vi "Memory Usage.vi"(8 "error in (no error)":errorcluster, 11 "System Status Actor in":refnum<class "System Status Actor.lvclass">) -> (0 "error out":errorcluster, 3 "System Status Actor out":refnum<class "System Status Actor.lvclass">)   [LabVIEW 2020, in "RTAF.lvlib" / "System Status Actor.lvclass"]
uses:
  System Status Actor.lvclass
  System Status Actor.lvclass/System Status Actor.ctl
panel:
  out "Total [MB]":dbl
  out "Used [MB]":dbl
  out "cat /proc/$(pidof lvrt)/status | grep RSS":string
  out "Free [MB]":dbl
  out "/proc/meminfo":string
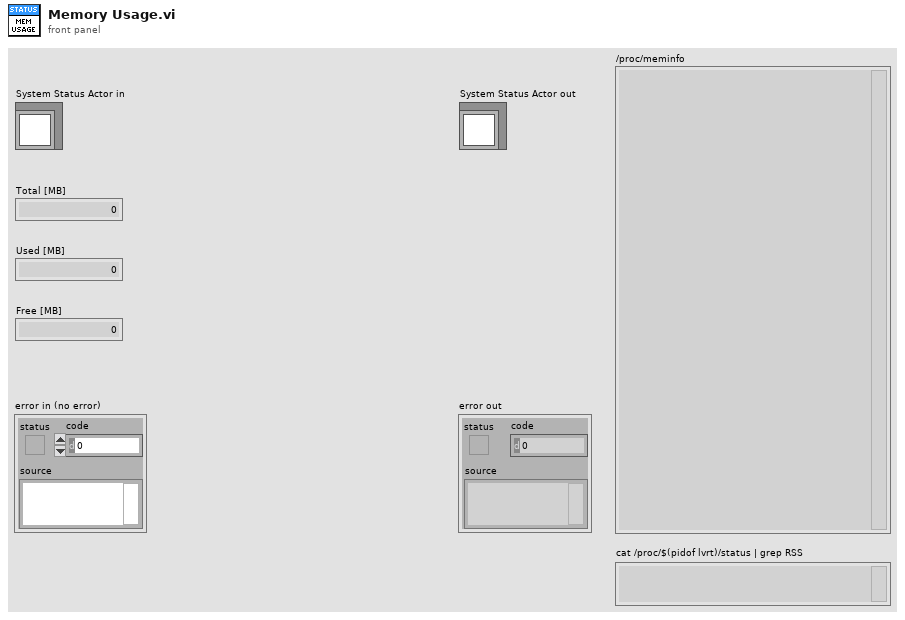
[diagram p1: front panel]
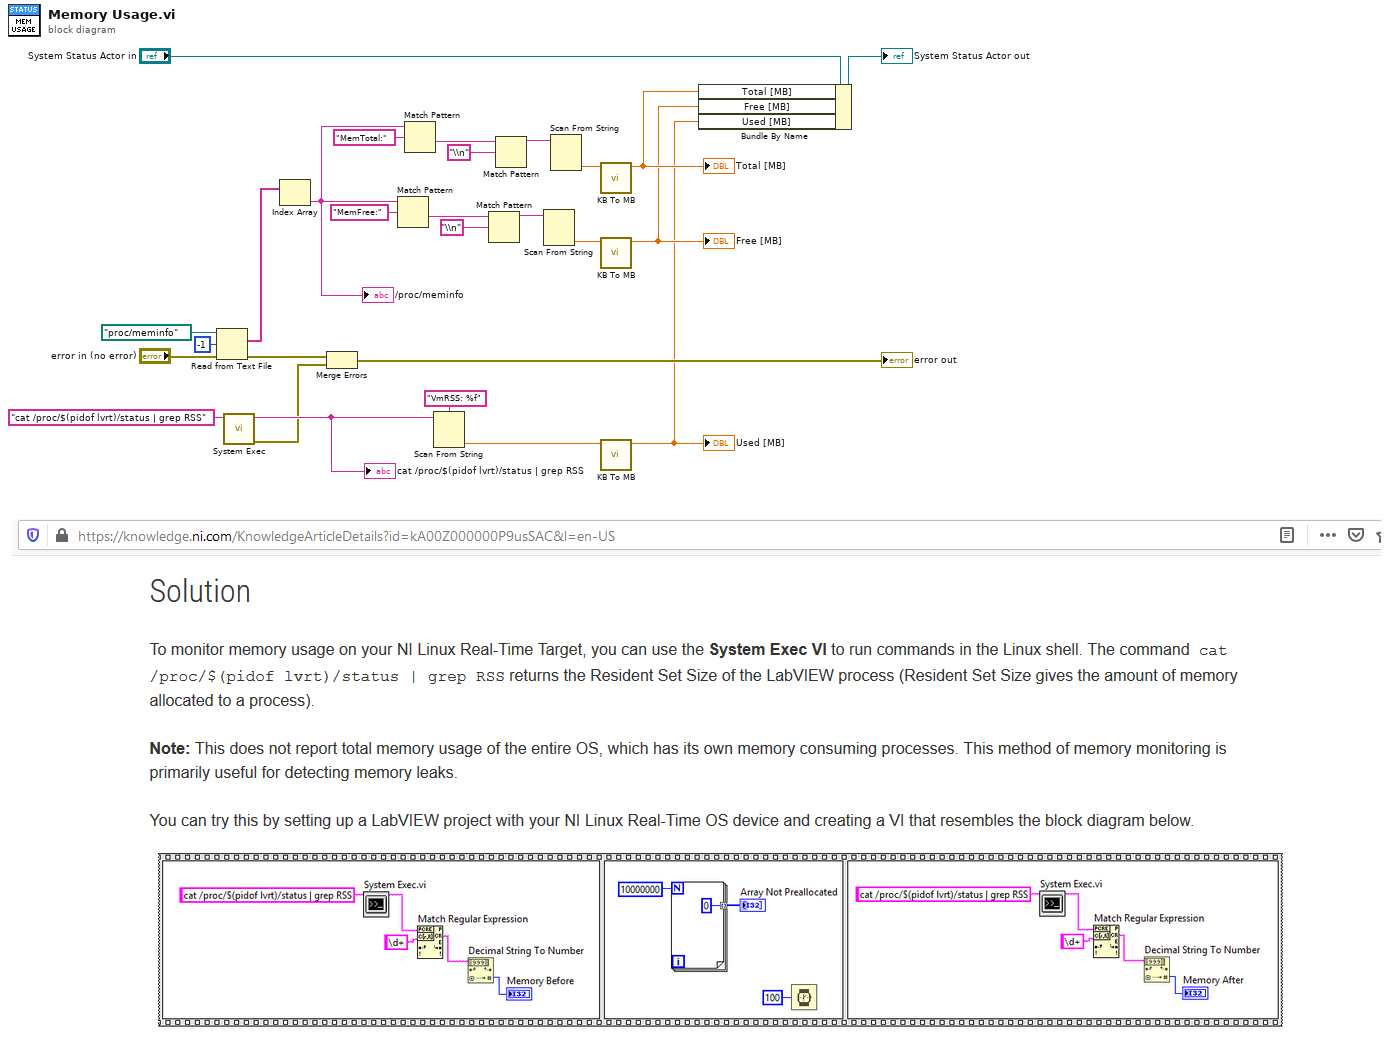
[diagram p0: block diagram]
diagram:
  n1 = Read from Text File(file (use dialog)=path "/proc/meminfo", count=-1, error in="error in (no error)") -> (text=w25:string[], error out=w17:errorcluster)  [unwired: 1 in, 2 out]
  n2 = call <vilib>:"System Exec.vi"("command line"="cat /proc/$(pidof lvrt)/status | grep RSS") -> ("error out"=w16:errorcluster, "standard output"=w19:string)  [unwired: 7 in, 2 out]
  "cat /proc/$(pidof lvrt)/status | grep RSS" <- w19
  n3 = Index Array(array=w25) -> (element=w11:string)  [unwired: 1 in]
  "/proc/meminfo" <- w11
  n4 = Merge Errors(w17, w16) -> (→"error out":errorcluster)
  n5 = Match Pattern(string=w11, regular expression="MemFree:") -> (after substring=w23:string)  [unwired: 1 in, 3 out]
  n6 = Match Pattern(string=w11, regular expression="MemTotal:") -> (after substring=w13:string)  [unwired: 1 in, 3 out]
  n7 = Scan From String(format string="VmRSS: %f", input string=w19) -> (output 1=w4:dbl)  [unwired: 3 in, 3 out]
  n8 = Match Pattern(string=w23, regular expression="\\n") -> (before substring=w21:string)  [unwired: 1 in, 3 out]
  n9 = Match Pattern(string=w13, regular expression="\\n") -> (before substring=w15:string)  [unwired: 1 in, 3 out]
  n10 = Scan From String(input string=w21) -> (output 1=w5:dbl)  [unwired: 4 in, 3 out]
  n11 = Scan From String(input string=w15) -> (output 1=w6:dbl)  [unwired: 4 in, 3 out]
  n12 = call "KB To MB.vi"("KB"=w6) -> ("MB"=w3:dbl)  [unwired: 10 in]
  "Total [MB]" <- w3
  n13 = call "KB To MB.vi"("KB"=w5) -> ("MB"=w2:dbl)  [unwired: 10 in]
  "Free [MB]" <- w2
  n14 = call "KB To MB.vi"("KB"=w4) -> ("MB"=w1:dbl)  [unwired: 10 in]
  "Used [MB]" <- w1
  n15 = Bundle By Name(cluster="System Status Actor in", "Total [MB]"=w3, "Free [MB]"=w2, "Used [MB]"=w1) -> (→"System Status Actor out":refnum<class "System Status Actor.lvclass">)
